vi "ConfigureCheckStepNameLength.vi"(0 "RuleConfigurationContext":refnum<k7>) -> (1 "status":bool, 2 "code":i32, 3 "source":string)   [LabVIEW 2011]
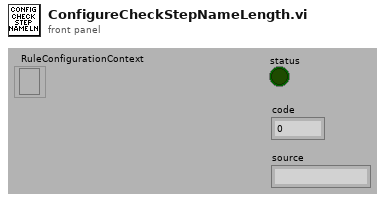
[diagram p1: front panel]
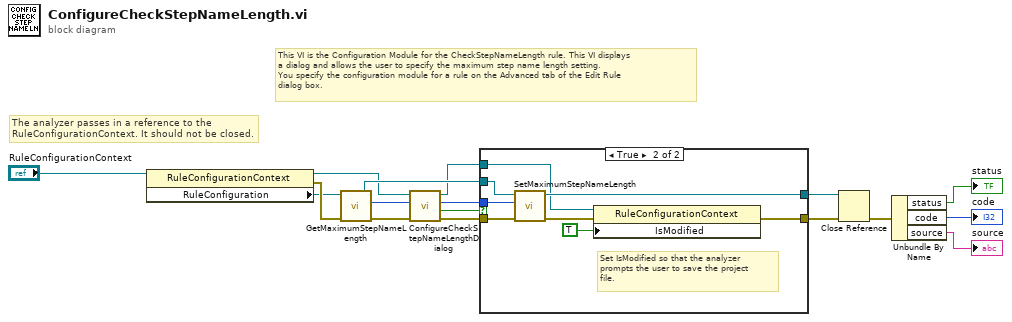
[diagram p0: block diagram]
diagram:
  # "The analyzer passes in a reference to the\nRuleConfigurationContext. It should not be closed."
  # "This VI is the Configuration Module for the CheckStepNameLength rule. This VI displays\na dialog and allows the user to specify the maximum step name length setting.\nYou specify the configuration module for a rule on the Advanced tab of the Edit Rule\ndialog box."
  n1 = property class="RuleConfigurationContext"(reference="RuleConfigurationContext") -> (reference out=w9:refnum<k7>, error out=w17:errorcluster, "RuleConfiguration"=w13:refnum<k7>)  [unwired: 1 in]
  n2 = call "GetMaximumStepNameLength.vi"("error in (no error)"=w17, "RuleConfiguration in"=w13) -> ("error out"=w10:errorcluster, "Maximum Step Name Length"=w8:i32, "RuleConfiguration out"=w16:refnum<k7>)  [unwired: 3 out]
  n3 = call "ConfigureCheckStepNameLengthDialog.vi"("error in (no error)"=w10, "Maximum Step Name Length:"=w8, "RuleConfigurationContext in"=w9) -> ("error out"=w14:errorcluster, "OKButtonClicked"=w5:bool, "Maximum Step Name Length out"=w7:i32, "RuleConfigurationContext out"=w6:refnum<k7>)  [unwired: 3 out]
  n4 = case shown="True" w5 {
    tunnel: w16 -> [w19 w27]
    tunnel: [w18 w25] -> w11
    tunnel: [w19 w24] -> w15
    tunnel: w14 -> [w18 w22]
    tunnel: w7 -> [_ w21]
    tunnel: w6 -> [_ w20]
    frame False {
    }
    frame True {
      # "Set IsModified so that the analyzer\nprompts the user to save the project\nfile."
      n5 = call "SetMaximumStepNameLength.vi"("error in (no error)"=w22, "Maximum Step Name Length"=w21, "RuleConfiguration in"=w27) -> ("error out"=w26:errorcluster, "RuleConfiguration out"=w24:refnum<k7>)  [unwired: 3 out]
      n6 = property class="RuleConfigurationContext"(reference=w20, error in=w26, "IsModified"=TRUE) -> (error out=w25:errorcluster)  [unwired: 1 out]
    }
  }
  n7 = Close Reference(reference=w15, error in (no error)=w11) -> (error out=w4:errorcluster)
  n8 = Unbundle By Name(w4) -> ("status"=→"status":bool, "code"=→"code":i32, "source"=→"source":string)
